vi "getNumFib.vi"(6 "Error":bool, 7 "VISA resource name":refnum<visa-resource-name>="ASRL13::INSTR") -> (0 "Fiber Count":i32, 2 "Error":bool, 3 "dup VISA resource name":refnum<visa-resource-name>="ASRL13::INSTR")   [LabVIEW 2018]
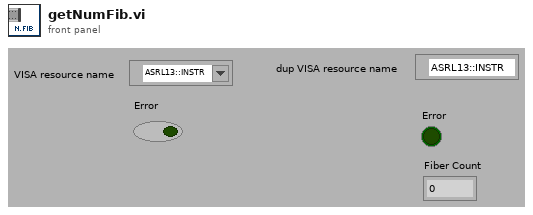
[diagram p1: front panel]
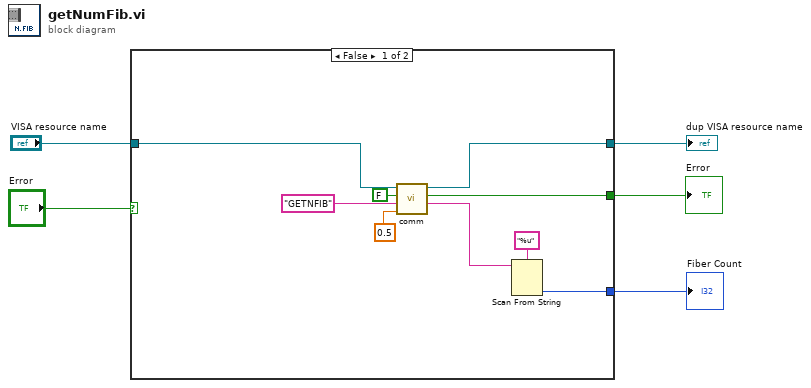
[diagram p0: block diagram]
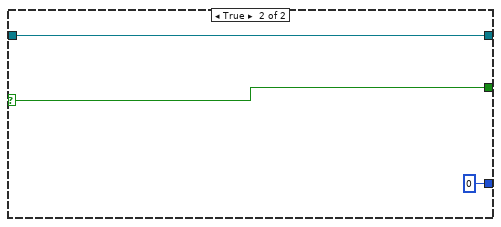
[diagram p2: hidden frame]
diagram:
  n1 = case shown="False" "Error" {
    selector: "Error" -> [_ w17]
    tunnel: "VISA resource name" -> [w14 w16]
    tunnel: [w9 w17] -> w4
    tunnel: [w13 w16] -> w3
    tunnel: [w6 u32 0] -> w1
    frame False {
      n2 = call "comm.vi"("Timeout (s)"=0.5, "Command"="GETNFIB", "Error"=FALSE, "VISA resource name"=w14) -> ("Response"=w7:string, "Error"=w9:bool, "dup VISA resource name"=w13:refnum<visa-resource-name>)  [unwired: 2 in, 1 out]
      n3 = Scan From String(format string="%u", input string=w7) -> (output 1=w6:u32)  [unwired: 3 in, 3 out]
    }
    frame True {
    }
  }
  "Error" <- w4
  "dup VISA resource name" <- w3
  "Fiber Count" <- w1
